vi "Create IgorColumnName.vi"(1 "X-Axis Unit":T1=enum."nm", 2 "FileName":string) -> (0 "Igor Column Names":string)   [LabVIEW 2019]
uses:
  Globals and TypeDefs/Type Definitions.llb/Wavelength Unit.ctt
  File and save/X-Axis Converter.llb/X-Axis Converter.vi
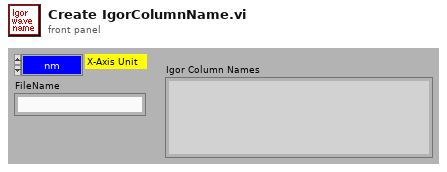
[diagram p1: front panel]
types:
  T1 = typedef "Wavelength Unit.ctt" = enum8{"Point", "nm", "eV", "meV", "cm_1"}
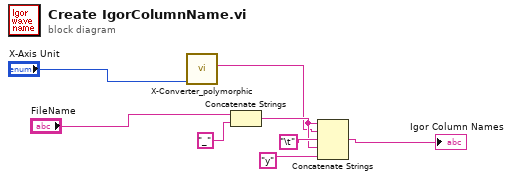
[diagram p0: block diagram]
diagram:
  n1 = call-poly "X-Converter_polymorphic.vi"("X-Axis Unit"="X-Axis Unit") -> ("X-Axis Unit String"=w4:string)  [unwired: 4 in, 3 out]
  n2 = Concatenate Strings("FileName", "_" ("string")) -> (w5:string)
  n3 = Concatenate Strings(w5, w4, "\t", w5, "y" ("string")) -> (→"Igor Column Names":string)
